vi "Looped TCP Read.vi"(7 "Server Alias":string, 8 "error in (no error)":errorcluster, 9 "timeout ms (25000)":i32, 10 "bytes to read":i32, 11 "connection ID in":refnum<k5>) -> (0 "error out":errorcluster, 2 "data out":string, 3 "connection ID out":refnum<k5>)   [LabVIEW 2013, in "TS.lvlib"]
doc: "Replaces normal TCP Read with an interruptible TCP Read that loops and polls the Stop global variable."
uses:
  TS.lvlib
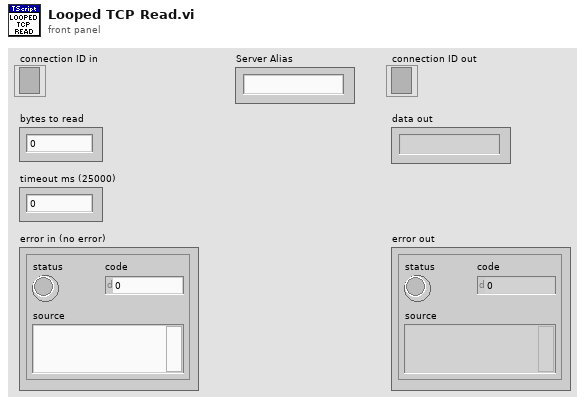
[diagram p1: front panel]
types:
  T1 = enum16{"Standard", "Buffered", "CRLF", "Immediate"}
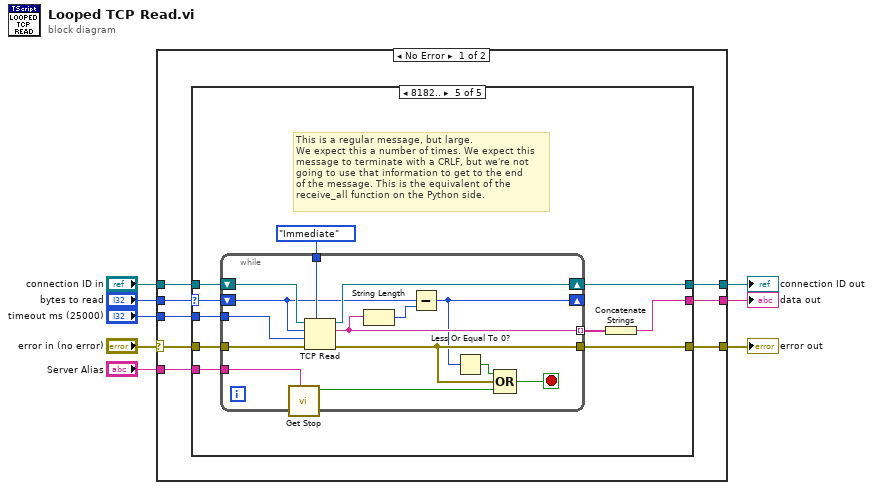
[diagram p0: block diagram]
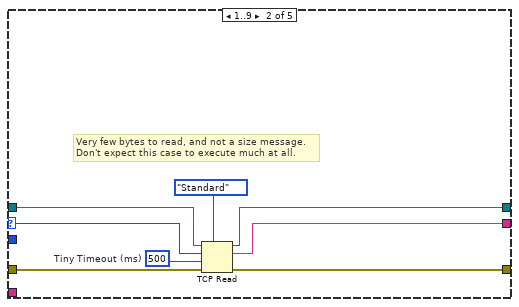
[diagram p3: hidden frame]
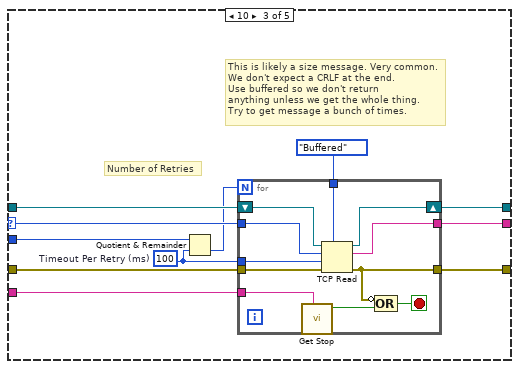
[diagram p4: hidden frame]
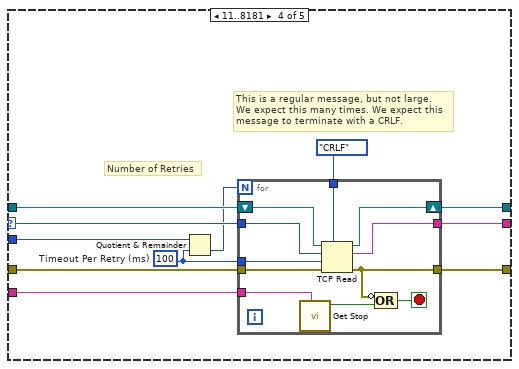
[diagram p5: hidden frame]
diagram:
  n1 = case shown="No Error" "error in (no error)" {
    selector: "error in (no error)" -> [w16 w95]
    tunnel: "connection ID in" -> [w14 w96]
    tunnel: "bytes to read" -> [w15 _]
    tunnel: [w13 w96] -> w6
    tunnel: [w12 w95] -> w4
    tunnel: [w11 _] -> w3
    tunnel: "timeout ms (25000)" -> [w10 _]
    tunnel: "Server Alias" -> [w9 _]
    frame No Error {
      n2 = case shown="8182.." w15 {
        selector: w15 -> [_ w25 w36 w58 w79]
        tunnel: w16 -> [w17 w26 w37 w59 w80]
        tunnel: w14 -> [w18 w24 w35 w57 w78]
        tunnel: [w18 w23 w34 w56 w77] -> w13
        tunnel: [w17 w21 w32 w54 w76] -> w12
        tunnel: [_ w22 w33 w55 w73] -> w11
        tunnel: w10 -> [_ _ w28 w50 w72]
        tunnel: w9 -> [_ _ w27 w49 w71]
        frame ..0 {
          # "Nothing to do. Skip."
        }
        frame 1..9 {
          w20 = 500  # Tiny Timeout (ms)
          # "Very few bytes to read, and not a size message.\nDon't expect this case to execute much at all."
          n3 = TCP Read(connection ID=w24, bytes to read=w25, error in (no error)=w26, 7:T1."Standard" ("mode (standard)"), 9:w20) -> (connection ID out=w23:refnum<k5>, data out=w22:string, error out=w21:errorcluster)
        }
        frame 10 {
          w29 = 100  # Timeout Per Retry (ms)
          # "Number of Retries"
          # "This is likely a size message. Very common.\nWe don't expect a CRLF at the end.\nUse buffered so we don't return \nanything unless we get the whole thing.\nTry to get message a bunch of times."
          n4 = Quotient & Remainder(x=w28, y=w29) -> (floor(x/y)=w30:i32)  [unwired: 1 out]
          n5 = for {
            N: w30 -> [_]
            tunnel: w36 -> [w47]
            tunnel: [w44] -> w33
            tunnel: T1."Buffered" ("mode (standard)") -> [w43]
            shift-right: [w45] -> w34
            shift-left: w35 -> [w46]
            tunnel: w37 -> [w48]
            tunnel: [w42] -> w32
            tunnel: w29 -> [w40]
            tunnel: w27 -> [w38]
            stop <- w41 stop-if-true
            n6 = call "Get Stop.vi"("Server Alias"=w38) -> ("Stop"=w39:bool)  [unwired: 9 in, 1 out]
            n7 = TCP Read(connection ID=w46, bytes to read=w47, error in (no error)=w48, 7:w43, 9:w40) -> (connection ID out=w45:refnum<k5>, data out=w44:string, error out=w42:errorcluster)
            n8 = Compound Arithmetic op=OR(invert w42, w39) -> (w41:bool)
          }
        }
        frame 11..8181 {
          w51 = 100  # Timeout Per Retry (ms)
          # "Number of Retries"
          # "This is a regular message, but not large.\nWe expect this many times. We expect this\nmessage to terminate with a CRLF."
          n9 = Quotient & Remainder(x=w50, y=w51) -> (floor(x/y)=w52:i32)  [unwired: 1 out]
          n10 = for {
            N: w52 -> [_]
            tunnel: w58 -> [w69]
            tunnel: [w66] -> w55
            tunnel: T1."CRLF" ("mode (standard)") -> [w65]
            shift-right: [w67] -> w56
            shift-left: w57 -> [w68]
            tunnel: w59 -> [w70]
            tunnel: [w64] -> w54
            tunnel: w51 -> [w62]
            tunnel: w49 -> [w60]
            stop <- w63 stop-if-true
            n11 = call "Get Stop.vi"("Server Alias"=w60) -> ("Stop"=w61:bool)  [unwired: 9 in, 1 out]
            n12 = TCP Read(connection ID=w68, bytes to read=w69, error in (no error)=w70, 7:w65, 9:w62) -> (connection ID out=w67:refnum<k5>, data out=w66:string, error out=w64:errorcluster)
            n13 = Compound Arithmetic op=OR(invert w64, w61) -> (w63:bool)
          }
        }
        frame 8182.. {
          # "This is a regular message, but large.\nWe expect this a number of times. We expect this\nmessage to terminate with a CRLF, but we're not\ngoing to use that information to get to the end\nof the message. This is the equivalent of the\nreceive_all function on the Python side."
          n14 = while {
            tunnel: [w89] -> w74 mode=indexing
            tunnel: T1."Immediate" ("mode (standard)") -> [w91]
            shift-right: [w92] -> w77
            shift-left: w78 -> [w93]
            tunnel: w80 -> [w94]
            tunnel: [w90] -> w76
            shift-right: [w86] -> _
            shift-left: w79 -> [w87]
            tunnel: w72 -> [w83]
            tunnel: w71 -> [w81]
            stop <- w84 stop-if-true
            n15 = call "Get Stop.vi"("Server Alias"=w81) -> ("Stop"=w82:bool)  [unwired: 9 in, 1 out]
            n16 = TCP Read(connection ID=w93, bytes to read=w87, error in (no error)=w94, 7:w91, 9:w83) -> (connection ID out=w92:refnum<k5>, data out=w89:string, error out=w90:errorcluster)
            n17 = String Length(string=w89) -> (length=w88:i32)
            n18 = Subtract(x=w87, y=w88) -> (x-y=w86:i32)
            n19 = Less Or Equal To 0?(x=w86) -> (x <= 0?=w85:bool)
            n20 = Compound Arithmetic op=OR(w85, w90, w82) -> (w84:bool)
          }
          n21 = Concatenate Strings(w74) -> (w73:string)
        }
      }
    }
    frame Error {
    }
  }
  "error out" <- w4
  "data out" <- w3
  "connection ID out" <- w6
